vi "subDCOffset.vi"(1 "Input signal samples":cdb[](array[numeric])) -> (0 "Output signal samples":cdb[](array[numeric]))   [LabVIEW 2012]
uses:
  <vilib>/Analysis/4window.llb/Hanning Window (DBL).vi
  <vilib>/Analysis/baseanly.llb/Mean (DBL).vi
  <vilib>/Analysis/NI_AALPro.lvlib
  <vilib>/Analysis/NI_AALBase.lvlib
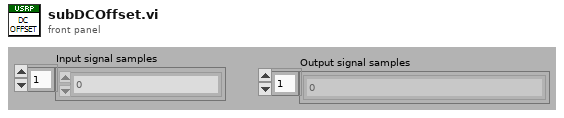
[diagram p1: front panel]
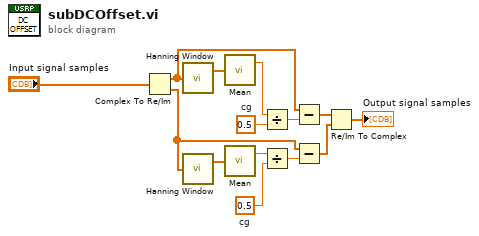
[diagram p0: block diagram]
diagram:
  w8 = 0.5  # cg
  w3 = 0.5  # cg
  n1 = Complex To Re/Im(x + iy="Input signal samples") -> (x=w10:dbl[], y=w11:dbl[])
  n2 = call-poly <vilib>:"Hanning Window.vi"("X"=w10) -> ("Windowed X"=w2:dbl[])  [unwired: 1 out]
  n3 = call-poly <vilib>:"Hanning Window.vi"("X"=w11) -> ("Windowed X"=w6:dbl[])  [unwired: 1 out]
  n4 = call-poly <vilib>:"Mean.vi"("X"=w2) -> ("mean"=w5:dbl)  [unwired: 1 out]
  n5 = call-poly <vilib>:"Mean.vi"("X"=w6) -> ("mean"=w9:dbl)  [unwired: 1 out]
  n6 = Divide(x=w5, y=w3) -> (x/y=w4:dbl)
  n7 = Divide(x=w9, y=w8) -> (x/y=w7:dbl)
  n8 = Subtract(x=w10, y=w4) -> (x-y=w13:dbl[])
  n9 = Subtract(x=w11, y=w7) -> (x-y=w14:dbl[])
  n10 = Re/Im To Complex(1:w14, 2:w13) -> (0:→"Output signal samples":cdb[])
